vi "runSettingsViewer.vi"(8 "error in (no error)":errorcluster, 11 "CameraManager.lvclass":refnum<class "CameraManager.lvclass">) -> (0 "error out":errorcluster)   [LabVIEW 2009, in "iManagement.lvlib" / "CameraManager.lvclass"]
uses:
  CameraManager.lvclass
  CameraManager.lvclass/CameraManager.ctl
  Hal/Channels/Camera/CameraController.lvclass
  Tools/SettingsViewer/settingsViewer.lvclass
  Tools/Filing/FileSystem/FileSystem.lvclass
  Hal/Channels/Camera/CameraEventsManager/CameraEventsManger.lvclass
  Tools/SettingsManager/SettingsManager.lvclass
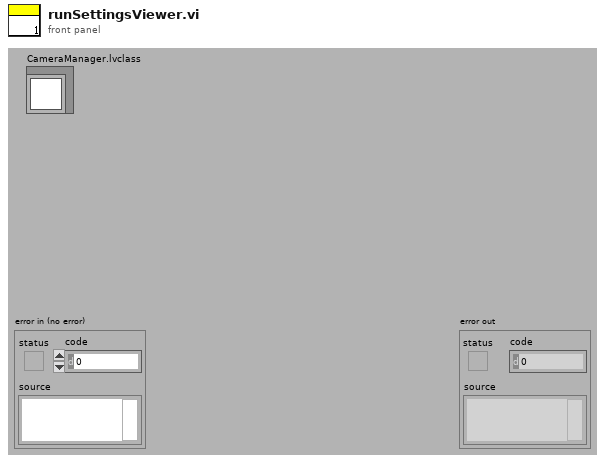
[diagram p1: front panel]
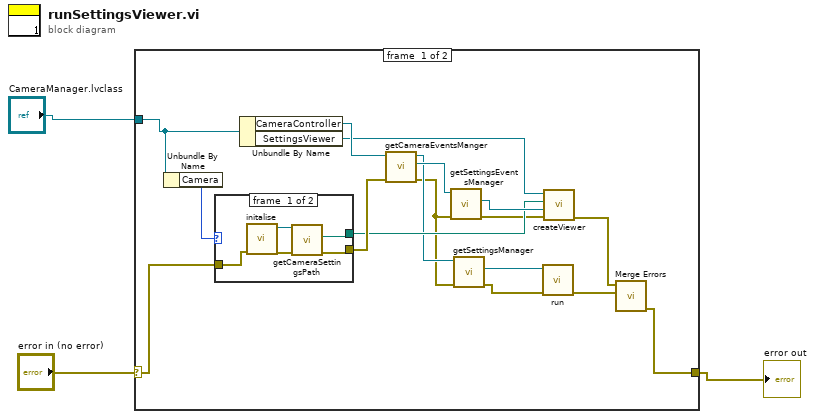
[diagram p0: block diagram]
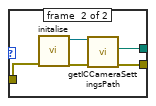
[diagram p2: hidden frame]
diagram:
  n1 = case shown="No Error" "error in (no error)" {
    selector: "error in (no error)" -> [w18 w31]
    tunnel: [w6 w31] -> w2
    tunnel: "CameraManager.lvclass" -> [w5 _]
    frame #0 {
      n2 = Unbundle By Name(w5) -> ("Camera"=w4:enum16{"AndorIKon", "ICCamera"})
      n3 = case shown="\"AndorIKon\", Default" w4 {
        tunnel: [w21 w28] -> w19
        tunnel: w18 -> [w25 w27]
        tunnel: [w22 w26] -> w16
        frame #0 {
          n4 = call "initalise.vi"("error in (no error)"=w25) -> ("error out"=w24:errorcluster, "FileSystem out"=w23:refnum<class "FileSystem.lvclass">)  [unwired: 9 in]
          n5 = call-dynamic "getCameraSettingsPath.vi"("error in (no error)"=w24, "FileSystem.lvclass in"=w23) -> ("error out"=w21:errorcluster, "CameraSettingsPath"=w22:path)  [unwired: 7 in, 1 out]
        }
        frame #1 {
          n6 = call "initalise.vi"("error in (no error)"=w27) -> ("error out"=w30:errorcluster, "FileSystem out"=w29:refnum<class "FileSystem.lvclass">)  [unwired: 9 in]
          n7 = call-dynamic "getICCameraSettingsPath.vi"("error in (no error)"=w30, "FileSystem.lvclass in"=w29) -> ("error out"=w28:errorcluster, "ICCameraSettingsPath"=w26:path)  [unwired: 7 in, 1 out]
        }
      }
      n8 = Unbundle By Name(w5) -> ("CameraController"=w20:refnum<class "CameraController.lvclass">, "SettingsViewer"=w15:refnum<class "settingsViewer.lvclass">)
      n9 = call-dynamic "getCameraEventsManger.vi"("error in (no error)"=w19, "CameraController.lvclass in"=w20) -> ("error out"=w11:errorcluster, "Hardware:Channels.lvlib:CameraEventsManger.lvclass"=w13:refnum<class "CameraEventsManger.lvclass">, "CameraController.lvclass out"=w12:refnum<class "CameraController.lvclass">)  [unwired: 7 in]
      n10 = call-dynamic "getSettingsEventsManager.vi"("error in (no error)"=w11, "CameraEventsManger.lvclass in"=w13) -> ("error out"=w14:errorcluster, "SettingsEventsManager"=w17:refnum<class "SettingsEventsManager.lvclass">)  [unwired: 7 in, 1 out]
      n11 = call-dynamic "getSettingsManager.vi"("error in (no error)"=w11, "CameraController.lvclass in"=w12) -> ("error out"=w10:errorcluster, "Tools.lvlib:Settings.lvlib:SettingsManager.lvclass"=w9:refnum<class "SettingsManager.lvclass">)  [unwired: 7 in, 1 out]
      n12 = call-dynamic "run.vi"("error in (no error)"=w10, "SettingsManager in"=w9) -> ("error out"=w7:errorcluster)  [unwired: 8 in, 1 out]
      n13 = call-dynamic "createViewer.vi"("error in (no error)"=w14, "SettingsEventsManager.lvclass"=w17, "Path"=w16, "Tools.lvlib:Settings.lvlib:SettingsViewer.lvclass"=w15) -> ("error out"=w8:errorcluster)  [unwired: 6 in, 1 out]
      n14 = call <vilib>:"Merge Errors.vi"("error in 2 (no error)"=w7, "error in 1 (no error)"=w8) -> ("error out"=w6:errorcluster)  [unwired: 5 in]
    }
    frame #1 {
    }
  }
  "error out" <- w2
